vi "Untitled controles.vi"() -> ()   [LabVIEW 2020]
panel:
  in  "Boolean 2":bool
  out "Numeric 3":dbl format="%#_13g"
  in  "Numeric 2":dbl format="%#_13g"
  in  "Numeric":dbl format="%#_13g"
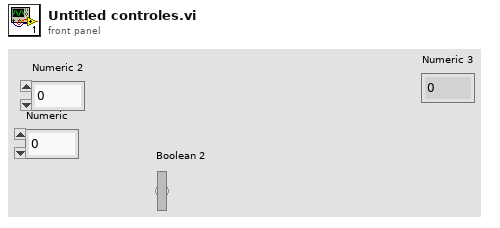
[diagram p1: front panel]
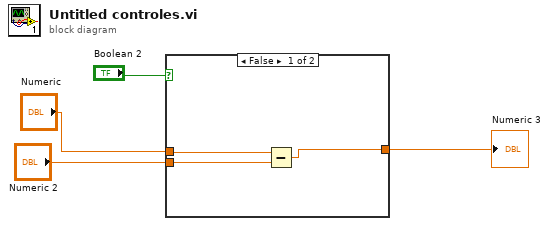
[diagram p0: block diagram]
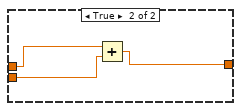
[diagram p2: hidden frame]
diagram:
  n1 = case shown="False" "Boolean 2" {
    tunnel: "Numeric" -> [w6 w10]
    tunnel: "Numeric 2" -> [w5 w9]
    tunnel: [w7 w8] -> w1
    frame False {
      n2 = Subtract(x=w6, y=w5) -> (x-y=w7:dbl)
    }
    frame True {
      n3 = Add(x=w10, y=w9) -> (x+y=w8:dbl)
    }
  }
  "Numeric 3" <- w1
